vi "过程变量.vi"() -> ()   [LabVIEW 2016, in "bbe.lvlib"]
uses:
  bbe.lvlib
panel:
  out "检测浓度":T1
  in  "BBE串口":refnum<visa-resource-name>
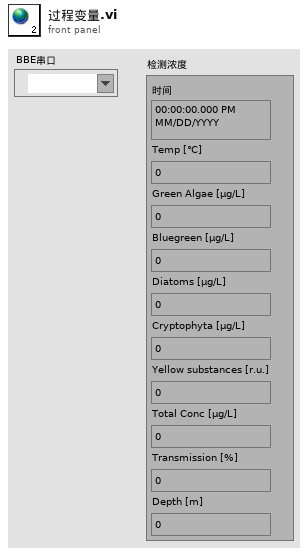
[diagram p1: front panel]
types:
  T1 = cluster{"时间":timestamp, "Temp [℃]":dbl, "Green Algae [μg/L]":dbl, "Bluegreen [μg/L]":dbl, "Diatoms [μg/L]":dbl, "Cryptophyta [μg/L]":dbl, "Yellow substances [r.u.]":dbl, "Total Conc [μg/L]":dbl, "Transmission [%]":dbl, "Depth [m]":dbl}
diagram:
